vi "Phasor Compute tau_phi & tau_m from Phasor (Continuous, Gated).vi"(8 "Error In":errorcluster, 9 "Phasor L_N[W] Parameters":T1, 11 "Phasor":cluster{"X":dbl, "Y":dbl}) -> (0 "Error Out":errorcluster, 1 "Modulus Lifetime":dbl[unit], 3 "Phase Lifetime":dbl[unit])   [LabVIEW 2021, in "Phasor.lvlib"]
uses:
  Phasor L_N[W] Parameters.ctl
  Phasor.lvlib
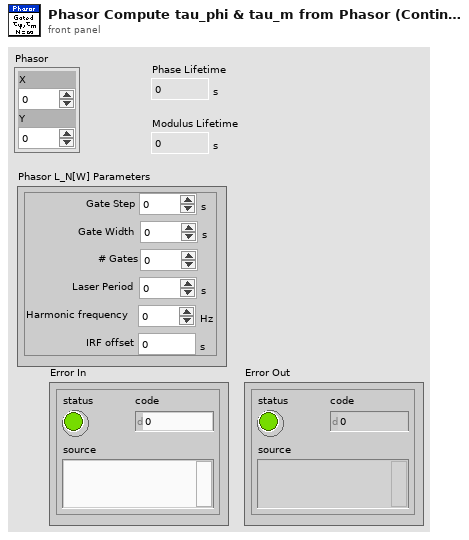
[diagram p1: front panel]
types:
  T1 = typedef "Phasor.lvlib/Phasor L_N[W] Parameters.ctl" = cluster{"Laser Period":dbl[unit], "Gate Width":dbl[unit], "Gate Step":dbl[unit], "Harmonic frequency":dbl[unit], "IRF offset":dbl[unit], "# Gates":dbl}
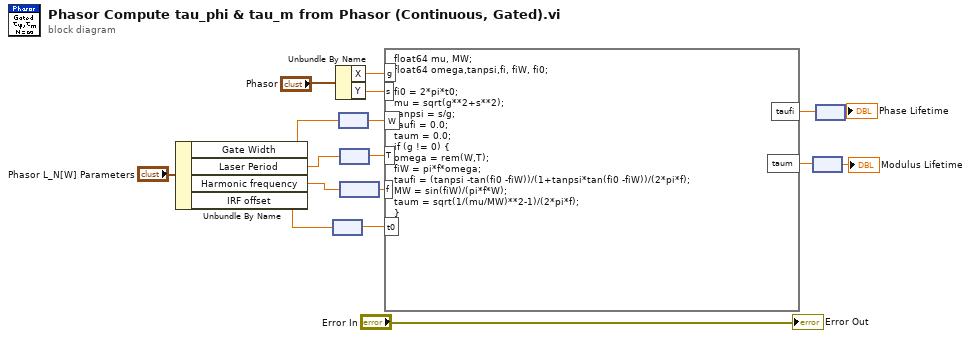
[diagram p0: block diagram]
diagram:
  n1 = Unbundle By Name("Phasor L_N[W] Parameters") -> ("Gate Width"=w5:dbl[unit], "Laser Period"=w4:dbl[unit], "Harmonic frequency"=w3:dbl[unit], "IRF offset"=w2:dbl[unit])
  n2 = node(w2) -> (w7:dbl)
  n3 = Unbundle By Name("Phasor") -> ("X"=w16:dbl, "Y"=w15:dbl)
  n4 = node(w5) -> (w14:dbl)
  n5 = node(w4) -> (w13:dbl)
  n6 = node(w3) -> (w12:dbl)
  n7 = formula code="float64 mu, MW;\nfloat64 omega,tanpsi,fi, fiW, fi0;\n\nfi0 = 2*pi*t0;\nmu = sqrt(g**2+s**2);\ntanpsi = s/g;\ntaufi = 0.0;\ntaum = 0.0;\nif (g != 0) {\nomega = rem(W,T);\nfiW = pi*f*omega;\ntaufi = (tanpsi -tan(fi0 -fiW))/(1+tanpsi*tan(fi0 -fiW))/(2*pi*f);\nMW = sin(fiW)/(pi*f*W);\ntaum = sqrt(1/(mu/MW)**2-1)/(2*pi*f);\n}"("g"=w16, "s"=w15, "W"=w14, "T"=w13, "f"=w12, "t0"=w7) -> ("taufi"=w11:dbl, "taum"=w9:dbl)
  n8 = node(w9) -> (→"Modulus Lifetime":dbl[unit])
  n9 = node(w11) -> (→"Phase Lifetime":dbl[unit])
  "Error Out" <- "Error In"
